vi "SC_schleife_T_control_init.vi"() -> ()   [LabVIEW 2019]
uses:
  Monitors/Utility/Monitor Communication/LS370/LS370-Control.ctl
  Global/Global Variables/global.vi
  Global/Global Variables/Data_Display_global.vi
  Instrument_Setup.vi
  Monitors/Utility/Monitor Communication/sub-vis/LS370_Open_Queue.vi
  <vilib>/Analysis/NI_AALBase.lvlib
  <vilib>/Analysis/NI_AALPro.lvlib
panel:
  out "Numeric 3":dbl format="%#_13g"
  out "Numeric 2":dbl format="%#_13g"
  out "XY Graph":T1(graph)
  out "Array":dbl[](array[numeric])
  out "Numeric":dbl format="%#_13g"
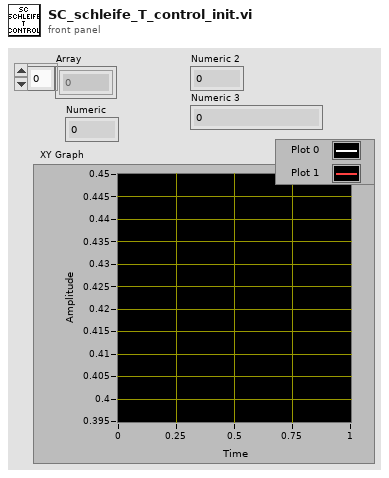
[diagram p1: front panel]
types:
  T1 = cluster{"Plot1":dbl[], "Best Linear Fit":dbl[]}[]
  T2 = typedef "LS370-Control.ctl" = cluster{"Disable Heater":bool, "Activate Tsweep":bool, "Update Lakeshores":bool, "Setpoint - Manual":dbl, "Rate (K/min)":dbl, "Sorb Power (mW)":dbl, "Still Power (mW)":dbl, "Sorb Heater":bool, "Still Heater":bool, "Set Temperature Sweep Main":bool}
  T3 = typedef "LS372-Cluster.ctl" = cluster{"Activate Tsweep":bool, "Setpoint - Manual":dbl, "Rate (K/min)":dbl, "Update Lakeshores":bool, "Still Heater":bool, "Still Power (mW)":dbl, "Manual Heater":bool, "Manual Heater  (mW) ":dbl, "Heater Range":dbl, "P (Gain)":dbl, "I (Reset)":dbl, "D (Rate)":dbl, "Heater Power (mW)":dbl, "MC Thermometer":u16, "MC Temperature":dbl, "LS372-T1":dbl, "LS372 -T2":dbl, "LS372-R1 ":dbl, "LS372-R2":dbl, "LS372-T3":dbl, "LS372-T4":dbl, "LS372-R3 ":dbl, "LS372-R4 \n\n\n\n":dbl, "LS372-T5":dbl, "LS372-T6":dbl, "LS372-R5":dbl, "LS372-R6 ":dbl, "Still Power ist":dbl, "Set Temperatur Sweep main":bool, "Setpoint ist":dbl, "Disable Heater":bool}
  T4 = typedef "Ls372-Control.ctl" = cluster{"Activate Tsweep":bool, "Setpoint - Manual":dbl, "Rate (K/min)":dbl, "Update Lakeshores":bool, "Still Heater":bool, "Still Power (mW)":dbl, "Manual Heater":bool, "Manual Heater  (mW) ":dbl, "MC Thermometer":u16, "Set Temperature Sweeep main":bool, "Disable Heater":bool}
  T5 = typedef "P9P14-TCluster.ctl" = cluster{"Setpoint":dbl, "Rate":dbl, "Chanel 1":dbl, "Approach":u16, "Set":bool, "Temperature\nStatus":i32, "Autoshutdown":bool}
  T6 = typedef "P9P14-TCluster-Control.ctl" = cluster{"Setpoint":dbl, "Rate":dbl, "Approach":u16, "Set":bool, "Autoshutdown":bool}
  T7 = typedef "ITC503Monitor-Cluster.ctl" = cluster{"Temperatur (K)":dbl, "Setpoint (K)":dbl, "Rate (K/min)":dbl, "Heater (%)":dbl, "NV (%)":dbl, "Heater Manual":bool, "NV Manual":bool, "Go to Set":bool, "Heater SP":dbl, "Valid?":bool, "Set Heater SP":bool, "Set NV SP":bool, "Heater (%) Display":dbl, "NV (%) Display":dbl, "NV Setpoint":dbl, "Change Heater Status":bool, "Change NV Status":bool, "Sample 3":dbl, "Sample 2":dbl, "Sweep-State":bool, "Set Auto PID":bool, "Auto PID":bool, "Stopp":bool, "Setpoint-Sweep":dbl, "Sample 1":dbl, "Control Channel":bool, "Channel 1":bool, "Channel 2":bool, "Channel 3":bool}
  T8 = typedef "ITC503_control.ctl" = cluster{"Setpoint (K)":dbl, "Rate (K/min)":dbl, "Go to Set":bool, "Set Heater SP":bool, "Set NV SP":bool, "Change Heater Status":bool, "Change NV Status":bool, "Set Auto PID":bool, "Stopp":bool, "Control Channel":bool, "Heater SP":dbl, "NV Setpoint":dbl}
  T9 = typedef "LS350-cluster.ctl" = cluster{"Setpoint":dbl, "Heater Output":dbl, "Setpoint control":dbl, "Enable Setpoint":bool, "LS350 T1":dbl, "LS350 T2":dbl, "LS350 T3":dbl, "LS350 T4":dbl, "LS350 R1":dbl, "LS350 R2":dbl, "LS350 R3":dbl, "LS350 R4":dbl}
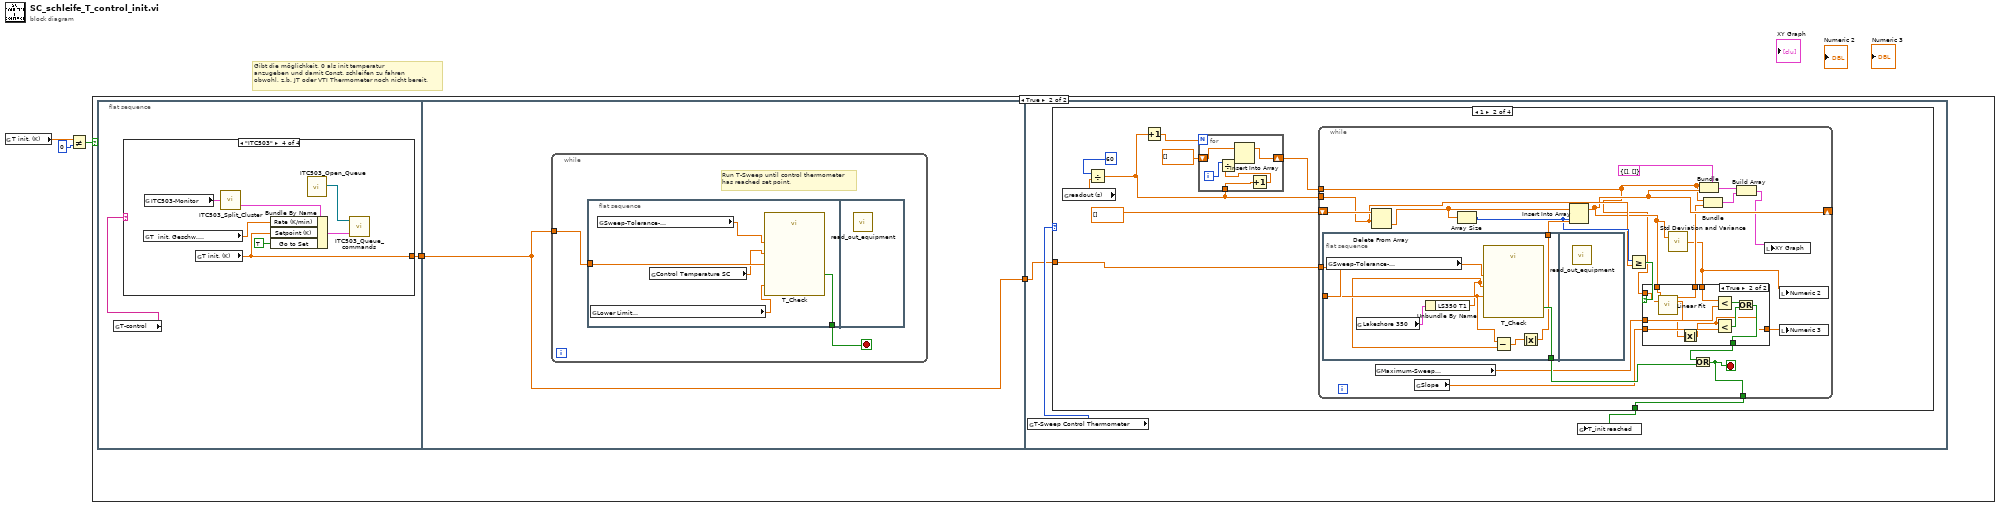
[diagram p0: block diagram]
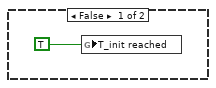
[diagram p2: hidden frame]
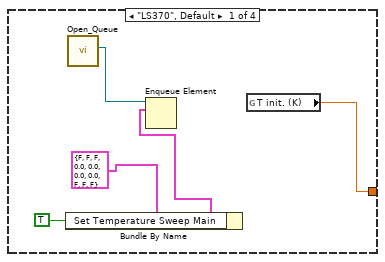
[diagram p3: hidden frame]
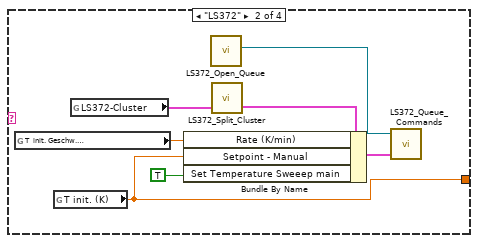
[diagram p4: hidden frame]
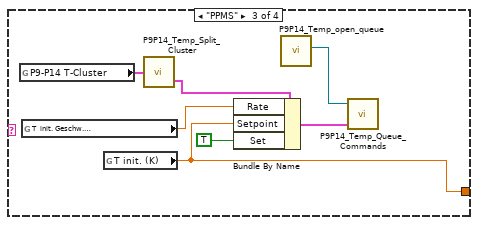
[diagram p5: hidden frame]
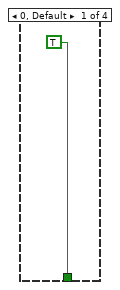
[diagram p6: hidden frame]
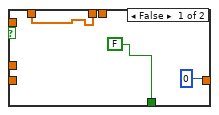
[diagram p7: hidden frame]
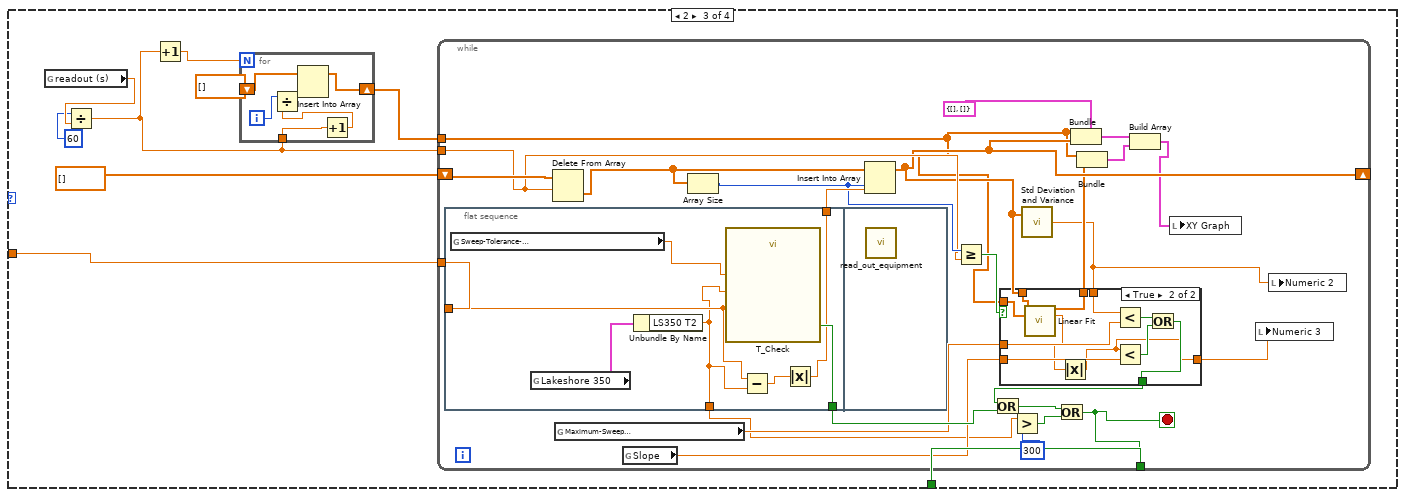
[diagram p8: hidden frame]
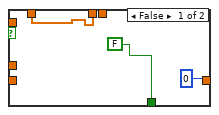
[diagram p9: hidden frame]
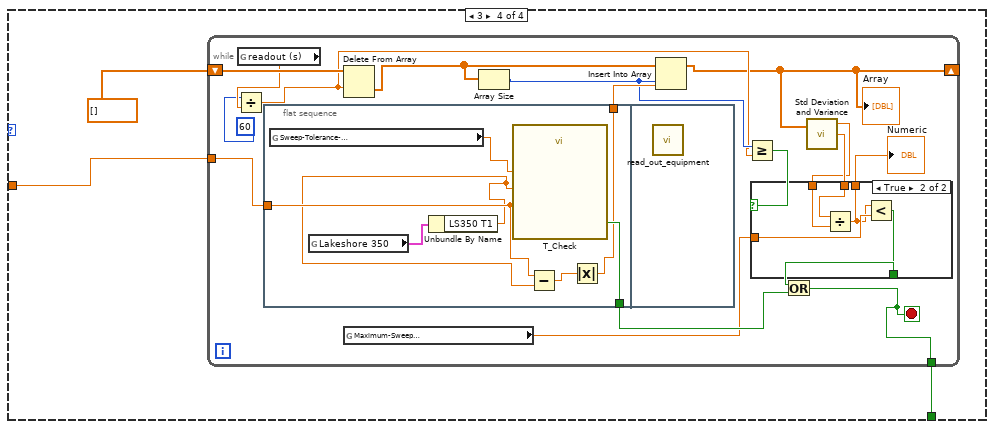
[diagram p10: hidden frame]
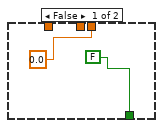
[diagram p11: hidden frame]
diagram:
  # "Gibt die möglichkeit, 0 als init temperatur \nanzugeben und damit Const. schleifen zu fahren\nobwohl, z.b. JT oder VTI Thermometer noch nicht bereit."
  n1 = global read "global.vi" "T init. (K)"() -> (w3:dbl)
  n2 = Not Equal?(x=w3, y=0) -> (x != y?=w1:bool)
  n3 = case shown="True" w1 {
    frame False {
      n4 = global write "Data_Display_global.vi" "T_init reached"(TRUE) -> ()
    }
    frame True {
      n5 = flat-sequence {
        tunnel: [w8] -> w6
        tunnel: w6 -> [w35]
        tunnel: [w35] -> w5
        tunnel: w5 -> [w44]
        frame #0 {
          n6 = global read "Instrument_Setup.vi" "T-control"() -> (w7:string)
          n7 = case shown="\"ITC503\"" w7 {
            tunnel: [w9 w14 w23 w28] -> w8
            frame "LS370", Default {
              n8 = Bundle By Name(cluster=T2 {"Disable Heater"=FALSE, "Activate Tsweep"=FALSE, "Update Lakeshores"=FALSE, "Setpoint - Manual"=0.0, "Rate (K/min)"=0.0, "Sorb Power (mW)"=0.0, "Still Power (mW)"=0.0, "Sorb Heater"=FALSE, "Still Heater"=FALSE, "Set Temperature Sweep Main"=FALSE} ("JT-Cluster"), "Set Temperature Sweep Main"=TRUE) -> (w10:T2)
              n9 = call-poly "Open_Queue.vi"() -> ("queue out"=w13:refnum<queue>)  [unwired: 10 in, 1 out]
              n10 = Enqueue Element(queue=w13, element=w10) -> ()  [unwired: 2 in, 3 out]
              n11 = global read "global.vi" "T init. (K)"() -> (w9:dbl)
            }
            frame "LS372" {
              n12 = global read "global.vi" "T  init. Geschw. \n(K/min)"() -> (w17:dbl)
              n13 = global read "global.vi" "T init. (K)"() -> (w14:dbl)
              n14 = global read "Data_Display_global.vi" "LS372-Cluster"() -> (w20:T3)
              n15 = call "LS372_Open_Queue.vi"() -> ("queue out"=w16:refnum<queue>)  [unwired: 10 in, 1 out]
              n16 = call "LS372_Split_Cluster.vi"("LS372-Cluster"=w20) -> ("LS372-Control"=w19:T4)  [unwired: 1 out]
              n17 = Bundle By Name(cluster=w19, "Rate (K/min)"=w17, "Setpoint - Manual"=w14, "Set Temperature Sweeep main"=TRUE) -> (w15:T4)
              n18 = call "LS372_Queue_Commands.vi"("LS372-Control"=w15, "Queue"=w16) -> ()  [unwired: 1 in, 1 out]
            }
            frame "PPMS" {
              n19 = global read "Data_Display_global.vi" "P9-P14 T-Cluster"() -> (w21:T5)
              n20 = global read "global.vi" "T  init. Geschw. \n(K/min)"() -> (w27:dbl)
              n21 = global read "global.vi" "T init. (K)"() -> (w23:dbl)
              n22 = call "P9P14_Temp_Split_Cluster.vi"("P9-P14 T-Cluster"=w21) -> ("P9-P14 T-Cluster -Control"=w22:T6)  [unwired: 1 out]
              n23 = Bundle By Name(cluster=w22, "Rate"=w27, "Setpoint"=w23, "Set"=TRUE) -> (w25:T6)
              n24 = call "P9P14_Temp_open_queue.vi"() -> ("queue out"=w26:refnum<queue>)  [unwired: 10 in, 1 out]
              n25 = call "P9P14_Temp_Queue_Commands.vi"("P9-P14 T-Cluster -Control"=w25, "Queue"=w26) -> ()  [unwired: 1 in, 1 out]
            }
            frame "ITC503" {
              n26 = global read "global.vi" "T  init. Geschw. \n(K/min)"() -> (w34:dbl)
              n27 = global read "Data_Display_global.vi" "ITC503-Monitor"() -> (w32:T7)
              n28 = global read "global.vi" "T init. (K)"() -> (w28:dbl)
              n29 = call "ITC503_Split_Cluster.vi"("ITC503-Monitor"=w32) -> ("ITC503-Control"=w31:T8)  [unwired: 1 out]
              n30 = Bundle By Name(cluster=w31, "Rate (K/min)"=w34, "Setpoint (K)"=w28, "Go to Set"=TRUE) -> (w30:T8)
              n31 = call "ITC503_Open_Queue.vi"() -> ("queue out"=w33:refnum<queue>)  [unwired: 10 in, 1 out]
              n32 = call "ITC503_Queue_commands.vi"("ITC503-Control"=w30, "ITC503 Queue"=w33) -> ()  [unwired: 1 in, 1 out]
            }
          }
        }
        frame #1 {
          n33 = while {
            tunnel: w35 -> [w37]
            stop <- w36 stop-if-true
            # "Run T-Sweep until control thermometer\nhas reached set point."
            n34 = flat-sequence {
              tunnel: w37 -> [w41]
              tunnel: [w42] -> w36
              frame #0 {
                n35 = global read "Instrument_Setup.vi" "Lower Limit\nSweep-Tolerance-\nTemperature (K)"() -> (w38:dbl)
                n36 = global read "Instrument_Setup.vi" "Sweep-Tolerance-\nTemperature (%)"() -> (w39:dbl)
                n37 = global read "Data_Display_global.vi" "Control Temperature SC"() -> (w40:dbl)
                n38 = call "T_Check.vi"("Lower Limit Sweep\nTolerance (K)"=w38, "T_target (K)"=w41, "Sweep\nTolerance %"=w39, "T_in"=w40) -> ("= T target"=w42:bool)
              }
              frame #1 {
                n39 = call "read_out_equipment.vi"() -> ()  [unwired: 1 in]
              }
            }
          }
        }
        frame #2 {
          n40 = global read "Instrument_Setup.vi" "T-Sweep Control Thermometer"() -> (w45:u16)
          n41 = case shown="1" w45 {
            tunnel: w44 -> [_ w54 w111 w166]
            tunnel: [TRUE w53 w110 w165] -> w43
            frame 0, Default {
            }
            frame 1 {
              n42 = global read "Instrument_Setup.vi" "readout (s)"() -> (w52:dbl)
              n43 = Divide(x=60, y=w52) -> (x/y=w48:dbl)
              n44 = Increment(x=w48) -> (x+1=w47:dbl)
              n45 = for {
                N: w47 -> [_]
                shift-right: [w58] -> w49
                shift-left: dbl[] [] -> [w61]
                tunnel: w48 -> [w57]
                i -> [w60]
                n46 = Increment(x=w57) -> (x+1=w56:dbl)
                n47 = Divide(x=w60, y=w56) -> (x/y=w59:dbl)
                n48 = Insert Into Array(array=w61, new element=w59) -> (w58:dbl[])  [unwired: 1 in]
              }
              n49 = while {
                tunnel: w54 -> [w82]
                shift-right: [w69] -> _
                shift-left: dbl[] [] -> [w81]
                tunnel: [w74] -> w53
                tunnel: w48 -> [w70]
                tunnel: w49 -> [w68]
                stop <- w74 stop-if-true
                n50 = flat-sequence {
                  tunnel: w82 -> [w101]
                  tunnel: [w98] -> w80
                  tunnel: [w102] -> w79
                  frame #0 {
                    n51 = global read "Instrument_Setup.vi" "Sweep-Tolerance-\nTemperature (%)"() -> (w103:dbl)
                    n52 = global read "Data_Display_global.vi" "Lakeshore 350"() -> (w97:T9)
                    n53 = Unbundle By Name(w97) -> ("LS350 T1"=w100:dbl)
                    n54 = call "T_Check.vi"("T_target (K)"=w101, "Sweep\nTolerance %"=w103, "T_in"=w100) -> ("= T target"=w102:bool)  [unwired: 1 in]
                    n55 = Subtract(x=w101, y=w100) -> (x-y=w99:dbl)
                    n56 = Absolute Value(x=w99) -> (abs(x)=w98:dbl)
                  }
                  frame #1 {
                    n57 = call "read_out_equipment.vi"() -> ()  [unwired: 1 in]
                  }
                }
                n58 = Delete From Array(array=w81, length=w70) -> (deleted portion=w77:dbl[])  [unwired: 1 in, 1 out]
                n59 = global read "Instrument_Setup.vi" "Maximum-Sweep\nSettle %/min"() -> (w75:dbl)
                n60 = global read "Instrument_Setup.vi" "Slope"() -> (w72:dbl)
                n61 = Array Size(array=w77) -> (size(s)=w71:i32)
                n62 = Insert Into Array(array=w77, index=w71, new element=w80) -> (w69:dbl[])
                n63 = Greater Or Equal?(x=w71, y=w70) -> (x >= y?=w76:bool)
                n64 = call <vilib>:"Std Deviation and Variance.vi"("X"=w69) -> ("standard deviation"=w63:dbl)  [unwired: 1 in, 2 out]
                n65 = case shown="True" w76 {
                  tunnel: w63 -> [_ w95]
                  tunnel: [FALSE w88] -> w78
                  tunnel: w75 -> [_ w96]
                  tunnel: w68 -> [_ w93]
                  tunnel: w69 -> [w84 w92]
                  tunnel: [w84 w91] -> w67
                  tunnel: w72 -> [_ w90]
                  tunnel: [0 w86] -> w64
                  frame False {
                  }
                  frame True {
                    n66 = call <vilib>:"Linear Fit.vi"("Y"=w92, "X"=w93) -> ("Best Linear Fit"=w91:dbl[], "slope"=w87:dbl)  [unwired: 9 in, 3 out]
                    n67 = Absolute Value(x=w87) -> (abs(x)=w86:dbl)
                    n68 = Less?(x=w95, y=w96) -> (x < y?=w94:bool)
                    n69 = Less?(x=w86, y=w90) -> (x < y?=w89:bool)
                    n70 = Or(x=w94, y=w89) -> (x .or. y?=w88:bool)
                  }
                }
                n71 = Or(x=w78, y=w79) -> (x .or. y?=w74:bool)
                n72 = Bundle(cluster=cluster{"Plot1":dbl[], "Plot 2":dbl[]} {"Plot1"=[], "Plot 2"=[]}, "Plot1"=w68, "Plot 2"=w69) -> (w66:cluster{"Plot1":dbl[], "Plot 2":dbl[]})
                n73 = Bundle(w68, "Best Linear Fit"=w67) -> (w65:cluster{dbl[], "Best Linear Fit":dbl[]})  [unwired: 1 in]
                n74 = Build Array(w66, w65) -> (w62:T1)
                n75 = local write "XY Graph"(w62) -> ()
                n76 = local write "Numeric 2"(w63) -> ()
                n77 = local write "Numeric 3"(w64) -> ()
              }
            }
            frame 2 {
              n78 = global read "Instrument_Setup.vi" "readout (s)"() -> (w109:dbl)
              n79 = Divide(x=60, y=w109) -> (x/y=w105:dbl)
              n80 = Increment(x=w105) -> (x+1=w104:dbl)
              n81 = for {
                N: w104 -> [_]
                shift-right: [w115] -> w106
                shift-left: dbl[] [] -> [w118]
                tunnel: w105 -> [w114]
                i -> [w117]
                n82 = Increment(x=w114) -> (x+1=w113:dbl)
                n83 = Divide(x=w117, y=w113) -> (x/y=w116:dbl)
                n84 = Insert Into Array(array=w118, new element=w116) -> (w115:dbl[])  [unwired: 1 in]
              }
              n85 = while {
                tunnel: w111 -> [w143]
                shift-right: [w131] -> _
                shift-left: dbl[] [] -> [w142]
                tunnel: [w119] -> w110
                tunnel: w105 -> [w132]
                tunnel: w106 -> [w130]
                stop <- w119 stop-if-true
                n86 = flat-sequence {
                  tunnel: w143 -> [w163]
                  tunnel: [w161] -> w141
                  tunnel: [w164] -> w140
                  tunnel: [w159] -> w123
                  frame #0 {
                    n87 = global read "Instrument_Setup.vi" "Sweep-Tolerance-\nTemperature (%)"() -> (w158:dbl)
                    n88 = global read "Data_Display_global.vi" "Lakeshore 350"() -> (w160:T9)
                    n89 = Unbundle By Name(w160) -> ("LS350 T2"=w159:dbl)
                    n90 = call "T_Check.vi"("T_target (K)"=w163, "Sweep\nTolerance %"=w158, "T_in"=w159) -> ("= T target"=w164:bool)  [unwired: 1 in]
                    n91 = Subtract(x=w163, y=w159) -> (x-y=w162:dbl)
                    n92 = Absolute Value(x=w162) -> (abs(x)=w161:dbl)
                  }
                  frame #1 {
                    n93 = call "read_out_equipment.vi"() -> ()  [unwired: 1 in]
                  }
                }
                n94 = Delete From Array(array=w142, length=w132) -> (deleted portion=w138:dbl[])  [unwired: 1 in, 1 out]
                n95 = global read "Instrument_Setup.vi" "Maximum-Sweep\nSettle %/min"() -> (w136:dbl)
                n96 = global read "Instrument_Setup.vi" "Slope"() -> (w134:dbl)
                n97 = Array Size(array=w138) -> (size(s)=w133:i32)
                n98 = Insert Into Array(array=w138, index=w133, new element=w141) -> (w131:dbl[])
                n99 = Greater Or Equal?(x=w133, y=w132) -> (x >= y?=w137:bool)
                n100 = Greater?(x=w123, y=300) -> (0:w121:bool)
                n101 = call <vilib>:"Std Deviation and Variance.vi"("X"=w131) -> ("standard deviation"=w125:dbl)  [unwired: 1 in, 2 out]
                n102 = case shown="True" w137 {
                  tunnel: w125 -> [_ w156]
                  tunnel: [FALSE w149] -> w139
                  tunnel: w136 -> [_ w157]
                  tunnel: w130 -> [_ w154]
                  tunnel: w131 -> [w145 w153]
                  tunnel: [w145 w152] -> w129
                  tunnel: w134 -> [_ w151]
                  tunnel: [0 w147] -> w124
                  frame False {
                  }
                  frame True {
                    n103 = call <vilib>:"Linear Fit.vi"("Y"=w153, "X"=w154) -> ("Best Linear Fit"=w152:dbl[], "slope"=w148:dbl)  [unwired: 9 in, 3 out]
                    n104 = Absolute Value(x=w148) -> (abs(x)=w147:dbl)
                    n105 = Less?(x=w156, y=w157) -> (x < y?=w155:bool)
                    n106 = Less?(x=w147, y=w151) -> (x < y?=w150:bool)
                    n107 = Or(x=w155, y=w150) -> (x .or. y?=w149:bool)
                  }
                }
                n108 = Or(x=w139, y=w140) -> (x .or. y?=w120:bool)
                n109 = Or(x=w120, y=w121) -> (x .or. y?=w119:bool)
                n110 = Bundle(cluster=cluster{"Plot1":dbl[], "Plot 2":dbl[]} {"Plot1"=[], "Plot 2"=[]}, "Plot1"=w130, "Plot 2"=w131) -> (w128:cluster{"Plot1":dbl[], "Plot 2":dbl[]})
                n111 = Bundle(w130, "Best Linear Fit"=w129) -> (w127:cluster{dbl[], "Best Linear Fit":dbl[]})  [unwired: 1 in]
                n112 = Build Array(w128, w127) -> (w126:T1)
                n113 = local write "XY Graph"(w126) -> ()
                n114 = local write "Numeric 3"(w124) -> ()
                n115 = local write "Numeric 2"(w125) -> ()
              }
            }
            frame 3 {
              n116 = while {
                tunnel: w166 -> [w184]
                shift-right: [w170] -> _
                shift-left: dbl[] [] -> [w183]
                tunnel: [w168] -> w165
                stop <- w168 stop-if-true
                n117 = global read "Instrument_Setup.vi" "readout (s)"() -> (w174:dbl)
                n118 = Divide(x=60, y=w174) -> (x/y=w172:dbl)
                n119 = flat-sequence {
                  tunnel: w184 -> [w197]
                  tunnel: [w194] -> w182
                  tunnel: [w198] -> w180
                  frame #0 {
                    n120 = global read "Instrument_Setup.vi" "Sweep-Tolerance-\nTemperature (%)"() -> (w192:dbl)
                    n121 = global read "Data_Display_global.vi" "Lakeshore 350"() -> (w193:T9)
                    n122 = Unbundle By Name(w193) -> ("LS350 T1"=w196:dbl)
                    n123 = call "T_Check.vi"("T_target (K)"=w197, "Sweep\nTolerance %"=w192, "T_in"=w196) -> ("= T target"=w198:bool)  [unwired: 1 in]
                    n124 = Subtract(x=w197, y=w196) -> (x-y=w195:dbl)
                    n125 = Absolute Value(x=w195) -> (abs(x)=w194:dbl)
                  }
                  frame #1 {
                    n126 = call "read_out_equipment.vi"() -> ()  [unwired: 1 in]
                  }
                }
                n127 = Delete From Array(array=w183, length=w172) -> (deleted portion=w178:dbl[])  [unwired: 1 in, 1 out]
                n128 = global read "Instrument_Setup.vi" "Maximum-Sweep\nSettle %/min"() -> (w171:dbl)
                n129 = Array Size(array=w178) -> (size(s)=w177:i32)
                n130 = Insert Into Array(array=w178, index=w177, new element=w182) -> (w170:dbl[])
                "Array" <- w170
                n131 = Greater Or Equal?(x=w177, y=w172) -> (x >= y?=w176:bool)
                n132 = call <vilib>:"Std Deviation and Variance.vi"("X"=w170) -> ("mean"=w175:dbl, "standard deviation"=w181:dbl)  [unwired: 1 in, 1 out]
                n133 = case shown="True" w176 {
                  tunnel: w181 -> [_ w191]
                  tunnel: [FALSE w189] -> w179
                  tunnel: w175 -> [_ w190]
                  tunnel: w171 -> [_ w188]
                  tunnel: [0.0 w187] -> w169
                  frame False {
                  }
                  frame True {
                    n134 = Divide(x=w191, y=w190) -> (x/y=w187:dbl)
                    n135 = Less?(x=w187, y=w188) -> (x < y?=w189:bool)
                  }
                }
                "Numeric" <- w169
                n136 = Or(x=w179, y=w180) -> (x .or. y?=w168:bool)
              }
            }
          }
          n137 = global write "Data_Display_global.vi" "T_init reached"(w43) -> ()
        }
      }
    }
  }
